vi "DCP Block Parser.vi"(8 "index":i32, 11 "Byte Array":u8[](array[numeric])) -> (0 "Block Last Byte":i32, 3 "Data":u8[](array[numeric]))   [LabVIEW 2017]
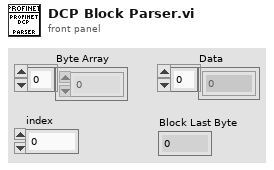
[diagram p1: front panel]
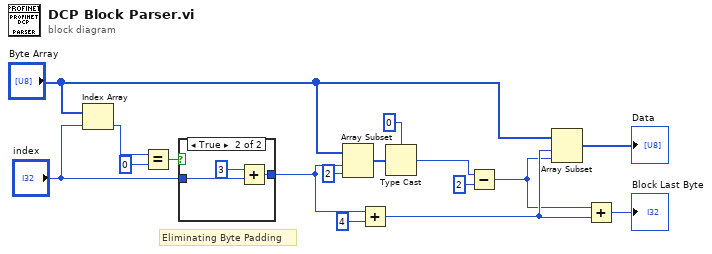
[diagram p0: block diagram]
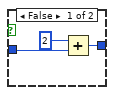
[diagram p2: hidden frame]
diagram:
  # "Eliminating Byte Padding"
  n1 = Index Array(array="Byte Array", index="index") -> (element=w2:u8)
  n2 = Equal?(x=w2, y=u8 0) -> (x = y?=w5:bool)
  n3 = case shown="True" w5 {
    tunnel: [w18 w22] -> w10
    tunnel: "index" -> [w17 w21]
    frame False {
      n4 = Add(x=2, y=w17) -> (x+y=w18:i32)
    }
    frame True {
      n5 = Add(x=3, y=w21) -> (x+y=w22:i32)
    }
  }
  n6 = Array Subset(array="Byte Array", index=w10, length=2) -> (w12:u8[])
  n7 = Add(x=w10, y=4) -> (x+y=w9:i32)
  n8 = Type Cast(type=u16 0, x=w12) -> (*(type *) &x=w14:u16)
  n9 = Subtract(x=w14, y=u8 2) -> (x-y=w8:u16)
  n10 = Array Subset(array="Byte Array", index=w9, length=w8) -> (→"Data":u8[])
  n11 = Add(x=w8, y=w9) -> (x+y=→"Block Last Byte":i32)
